vi "Compile Communication Configuration.vi"(8 "error in (no error)":errorcluster, 11 "Device Ref in":T1 format="%.0x") -> (0 "error out":errorcluster, 2 "Communication Configuration":T2, 3 "Device Ref out":T1 format="%.0x")   [LabVIEW 2020, in "Routing and Faulting System Explorer.lvlib"]
uses:
  Routing and Faulting System Explorer.lvlib
  Shared/Communication Configuration.ctl
  <vilib>/NI VeriStand/Custom Device API/Custom Device Item Ref.ctl
  Shared/Routing and Faulting Shared.lvlib
  <vilib>/NI VeriStand/Custom Device API/Custom Device API.lvlib
  Shared/Routing and Faulting Hardware API/Routing and Faulting Hardware API.lvlib
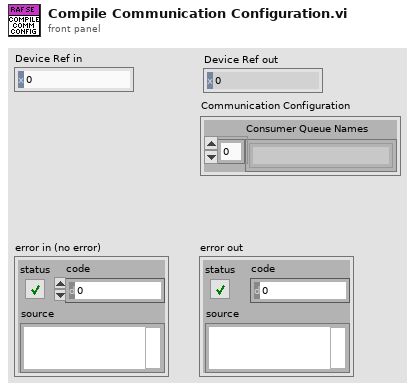
[diagram p1: front panel]
types:
  T1 = typedef "Custom Device API.lvlib/Custom Device Item Ref.ctl" = u64
  T2 = typedef "Routing and Faulting Shared.lvlib/Communication Configuration.ctl" = cluster{"Consumer Queue Names":string[]}
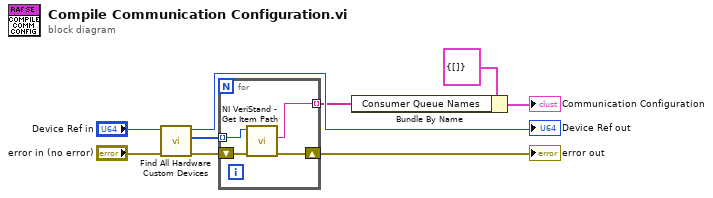
[diagram p0: block diagram]
diagram:
  n1 = call "Find All Hardware Custom Devices.vi"("error in (no error)"="error in (no error)", "Routing and Faulting Ref in"="Device Ref in") -> ("error out"=w5:errorcluster, "Hardware Refs"=w2:T1[], "Routing and Faulting Ref out"=→"Device Ref out":T1)  [unwired: 7 in]
  n2 = for {
    shift-right: [w11] -> w4
    shift-left: w5 -> [w13]
    tunnel: w2 -> [w12] mode=indexing
    tunnel: [w10] -> w1 mode=indexing
    n3 = call <vilib>:"NI VeriStand - Get Item Path.vi"("error in (no error)"=w13, "Item Ref in"=w12) -> ("error out"=w11:errorcluster, "Path"=w10:string)  [unwired: 6 in, 2 out]
  }
  "error out" <- w4
  n4 = Bundle By Name(cluster=T2 {"Consumer Queue Names"=[]} ("Communication Configuration 2"), "Consumer Queue Names"=w1) -> (→"Communication Configuration":T2)
